vi "SendCmd.vi"(6 "Comment":string, 8 "Add Chksm":bool=TRUE, 9 "Array In":u8[](array[numeric]), 11 "Python in":string) -> (1 "Array Sent":u8[](array[numeric]), 3 "Python out":string)   [LabVIEW 2016]
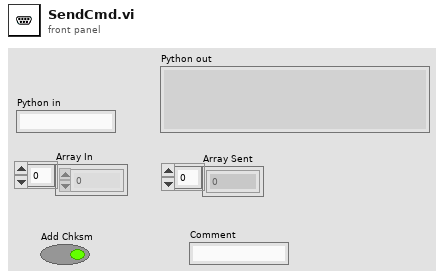
[diagram p1: front panel]
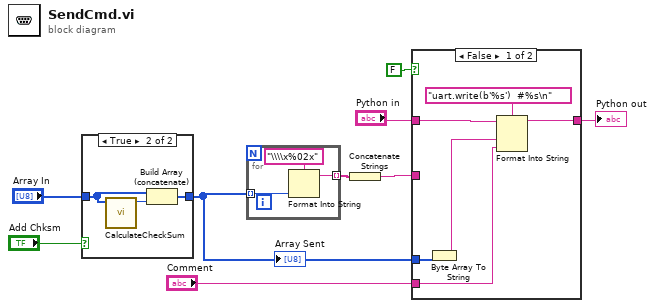
[diagram p0: block diagram]
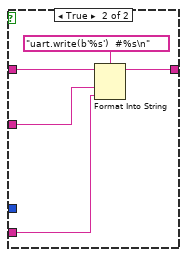
[diagram p2: hidden frame]
diagram:
  n1 = case shown="True" "Add Chksm" {
    tunnel: "Array In" -> [w10 w12]
    tunnel: [w10 w11] -> w2
    frame False {
    }
    frame True {
      n2 = call "CalculateCheckSum.vi"("Array"=w12) -> ("checksum"=w13:u8)  [unwired: 10 in]
      n3 = Build Array (concatenate)(w12, w13) -> (w11:u8[])
    }
  }
  "Array Sent" <- w2
  n4 = for {
    tunnel: w2 -> [w15] mode=indexing
    tunnel: [w14] -> w6 mode=indexing
    n5 = Format Into String(format string="\\\\x%02x", w15) -> (resulting string=w14:string)  [unwired: 2 in, 1 out]
  }
  n6 = Concatenate Strings(w6) -> (w5:string)
  n7 = case shown="False" FALSE {
    tunnel: "Python in" -> [w21 w26]
    tunnel: [w20 w25] -> w7
    tunnel: w5 -> [_ w24]
    tunnel: w2 -> [w22 _]
    tunnel: "Comment" -> [w18 w23]
    frame False {
      n8 = Byte Array To String(unsigned byte array=w22) -> (string=w19:string)
      n9 = Format Into String(format string="uart.write(b'%s')  #%s\n", initial string=w21, w19, w18) -> (resulting string=w20:string)  [unwired: 1 in, 1 out]
    }
    frame True {
      n10 = Format Into String(format string="uart.write(b'%s')  #%s\n", initial string=w26, w24, w23) -> (resulting string=w25:string)  [unwired: 1 in, 1 out]
    }
  }
  "Python out" <- w7
